vi "Report.vi"(6 "文件重命名":bool, 7 "文件名称":string, 8 "错误输入（无错误）":errorcluster, 11 "检测结果":bool[][](array[boolean])=[[TRUE]]) -> (0 "error out":errorcluster caption="错误输出", 3 "PRODUCT_VAULE":string)   [LabVIEW 2020]
uses:
  Global_Variable/Global.vi
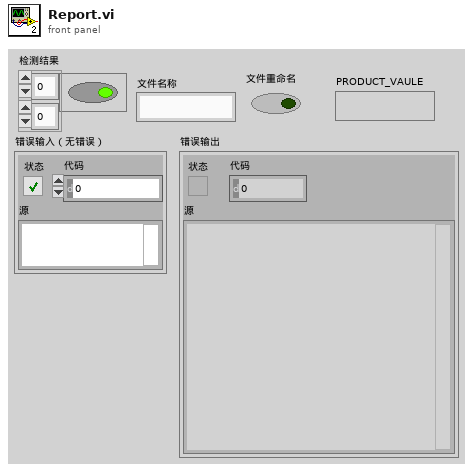
[diagram p1: front panel]
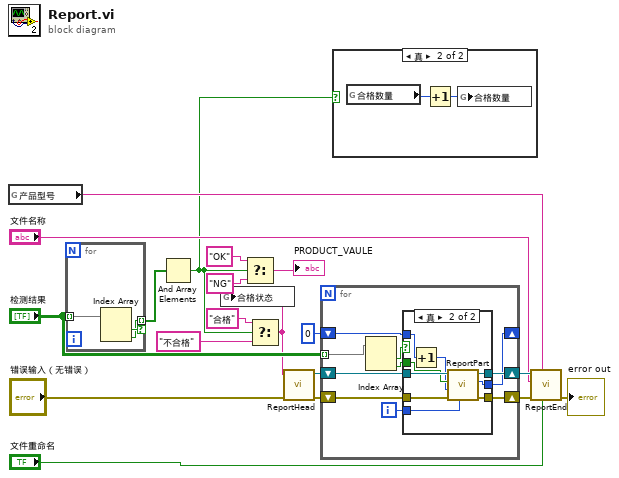
[diagram p0: block diagram]
diagram:
  n1 = global read "Global.vi" "产品型号"() -> (w3:string)
  n2 = for {
    tunnel: [w20] -> w6 mode=indexing if=w21
    tunnel: "检测结果" -> [w22] mode=indexing
    n3 = Index Array(array=w22) -> (element #1=w21:bool, element #2=w20:bool)  [unwired: 2 in]
  }
  n4 = And Array Elements(Boolean array=w6) -> (logical AND=w1:bool)
  n5 = Select(t="OK", s=w1, f="NG") -> (s? t:f=→"PRODUCT_VAULE":string)
  n6 = Select(t="合格", s=w1, f="不合格") -> (s? t:f=w2:string)
  n7 = global write "检测结果.vi" "合格状态"(w2) -> ()
  n8 = call "ReportHead.vi"("error in (no error)"="错误输入（无错误）", "产品状态"=w2) -> ("error out"=w18:errorcluster, "report out"=w19:refnum<class "NI_report.lvclass">)  [unwired: 8 in]
  n9 = for {
    shift-right: [w30] -> w17
    shift-left: w19 -> [w32]
    shift-right: [w29] -> w16
    shift-left: w18 -> [w31]
    tunnel: "检测结果" -> [w25] mode=indexing
    shift-right: [w26] -> _
    shift-left: 0 ("索引OUT") -> [w27]
    i -> [w28]
    n10 = Index Array(array=w25) -> (element #1=w24:bool, element #2=w23:bool)  [unwired: 2 in]
    n11 = case shown="真" w24 {
      tunnel: w32 -> [w34 w44]
      tunnel: w31 -> [w35 w43]
      tunnel: [w34 w42] -> w30
      tunnel: [w35 w41] -> w29
      tunnel: w28 -> [_ w40]
      tunnel: w23 -> [_ w39]
      tunnel: w27 -> [w33 w37]
      tunnel: [w33 w38] -> w26
      frame False {
      }
      frame True {
        n12 = Increment(x=w37) -> (x+1=w36:i32)
        n13 = call "ReportPart.vi"("试验项目"=w40, "error in"=w43, "索引IN"=w36, "合格"=w39, "report in"=w44) -> ("error out 2"=w41:errorcluster, "索引OUT"=w38:i32, "report out"=w42:refnum<class "NI_report.lvclass">)  [unwired: 4 in]
      }
    }
  }
  n14 = case shown="真" w1 {
    frame False {
    }
    frame True {
      n15 = global read "Global.vi" "合格数量"() -> (w46:i32)
      n16 = Increment(x=w46) -> (x+1=w45:i32)
      n17 = global write "Global.vi" "合格数量"(w45) -> ()
    }
  }
  n18 = call "ReportEnd.vi"("文件重命名"="文件重命名", "产品型号"=w3, "error in (no error)"=w16, "文件名称"="文件名称", "report in"=w17) -> ("error out"=→"error out":errorcluster)  [unwired: 6 in]
